vi "getTimeChannelFromXmlNative.vi"(8 "error in (no error)":errorcluster, 10 "eventXML":refnum<k20>, 11 "ScriptEvent in":refnum<class "ScriptEvent.lvclass">) -> (0 "error out":errorcluster, 2 "eventXML out":refnum<k20>, 3 "ScriptEvent out":refnum<class "ScriptEvent.lvclass">)   [LabVIEW 2011, in "Tools.lvlib" / "Scripting.lvlib" / "ScriptEvent.lvclass"]
uses:
  ScriptEvent.lvclass
  DatabaseHelpers/Database Objects/Channel/Channel.lvclass
  <vilib>/xml/Close Reference(Node).vi
  <vilib>/xml/Close Reference(NNMap).vi
  Program Files/National Instruments/LabVIEW 2011/resource/objmgr/DOMUserDefRef.rc
  <vilib>/xml/NI_XML.lvlib
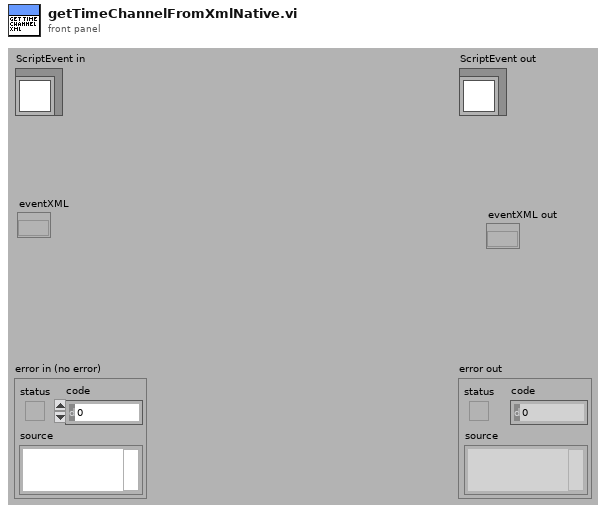
[diagram p1: front panel]
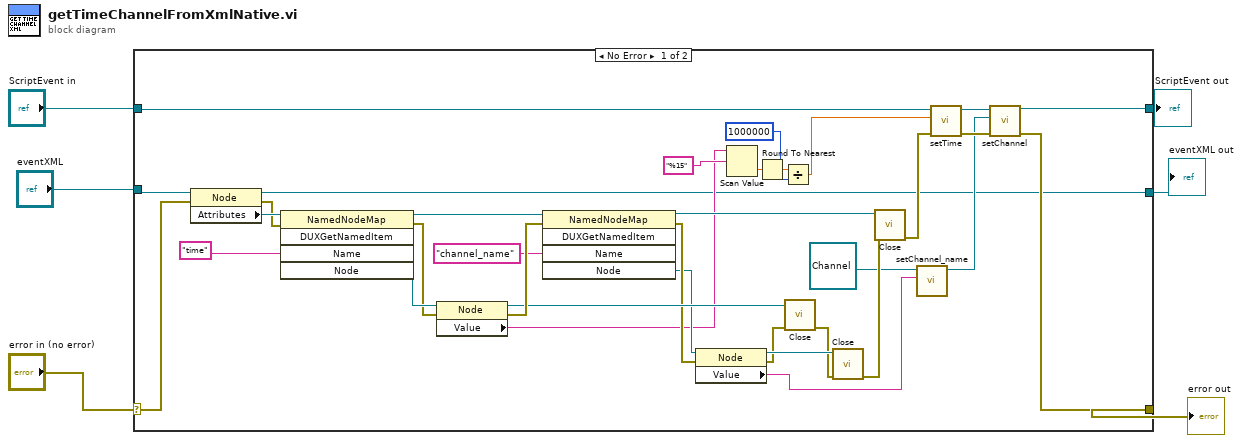
[diagram p0: block diagram]
diagram:
  n1 = case shown="No Error" "error in (no error)" {
    selector: "error in (no error)" -> [w14 w42]
    tunnel: [w15 w42] -> w5
    tunnel: [w16 w41] -> w3
    tunnel: "ScriptEvent in" -> [w17 w41]
    tunnel: "eventXML" -> [w40 _]
    tunnel: [w8 _] -> w1
    frame No Error {
      n2 = property class="Node"(reference=w40, error in=w14) -> (reference out=w8:refnum<k20>, error out=w36:errorcluster, "Attributes"=w37:refnum<k20>)
      n3 = invoke class="NamedNodeMap" method="DUXGetNamedItem"(reference=w37, error in=w36, "Name"="time") -> (reference out=w35:refnum<k20>, error out=w38:errorcluster, "Node"=w39:refnum<k20>)  [unwired: 2 in, 2 out]
      n4 = property class="Node"(reference=w39, error in=w38) -> (reference out=w33:refnum<k20>, error out=w34:errorcluster, "Value"=w22:string)
      n5 = invoke class="NamedNodeMap" method="DUXGetNamedItem"(reference=w35, error in=w34, "Name"="channel_name") -> (reference out=w28:refnum<k20>, error out=w27:errorcluster, "Node"=w26:refnum<k20>)  [unwired: 2 in, 2 out]
      n6 = property class="Node"(reference=w26, error in=w27) -> (reference out=w32:refnum<k20>, error out=w31:errorcluster, "Value"=w10:string)
      n7 = Scan Value(string=w22, format string="%15") -> (value=w21:dbl)  [unwired: 1 in, 1 out]
      n8 = Round To Nearest(number=w21) -> (nearest integer value=w7:dbl)
      n9 = Divide(x=w7, y=1000000) -> (x/y=w13:dbl)
      n10 = call-poly <vilib>:"Close.vi"("error in (no error)"=w31, "node"=w33) -> ("error out"=w30:errorcluster)  [unwired: 7 in]
      n11 = call-poly <vilib>:"Close.vi"("error in (no error)"=w30, "node"=w32) -> ("error out"=w29:errorcluster)  [unwired: 7 in]
      n12 = call-poly <vilib>:"Close.vi"("error in (no error)"=w29, "named node map"=w28) -> ("error out"=w12:errorcluster)  [unwired: 7 in]
      n13 = call "setChannel_name.vi"("channel_name"=w10, "Channel.lvclass in"=refnum<class "Channel.lvclass"> refnum ("Tools.lvlib:DatabaseHelpers.lvlib:Channel.lvclass")) -> ("Channel.lvclass out"=w9:refnum<class "Channel.lvclass">)  [unwired: 8 in, 1 out]
      n14 = call "setTime.vi"("error in (no error)"=w12, "time"=w13, "ScriptEvent.lvclass in"=w17) -> ("error out"=w18:errorcluster, "ScriptEvent.lvclass out"=w19:refnum<class "ScriptEvent.lvclass">)  [unwired: 7 in]
      n15 = call-dynamic "setChannel.vi"("error in (no error)"=w18, "Channel.lvclass"=w9, "ScriptEvent.lvclass in"=w19) -> ("error out"=w15:errorcluster, "ScriptEvent.lvclass out"=w16:refnum<class "ScriptEvent.lvclass">)  [unwired: 7 in]
    }
    frame Error {
    }
  }
  "error out" <- w5
  "ScriptEvent out" <- w3
  "eventXML out" <- w1
